vi "ShortcutMenu.vi"(8 "error in":errorcluster, 9 "menu ref in":refnum<k9>, 11 "node in":refnum<class "NISE_CEF_Node.lvclass">) -> (0 "error out":errorcluster, 1 "menu ref out":refnum<k9>, 3 "node out":refnum<class "NISE_CEF_Node.lvclass">)   [LabVIEW 2013, in "NISE_CEF_Node.lvclass"]
doc: "Defines the behavior of the shortcut menu of the node."
uses:
  NISE_CEF_Node.lvclass
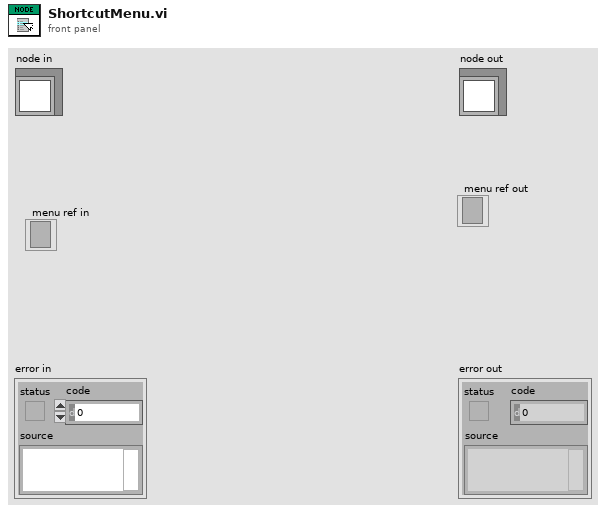
[diagram p1: front panel]
types:
  T1 = typedef "NISE_CEF_Node.lvclass/NodeMenuOptions.ctl" = cluster{"removable":bool, "movable":bool, "duplicate":bool}
  T2 = typedef "NISE_CEF_Node.lvclass/SubNodeCluster.ctl" = cluster{"subnodes menu name":string[], "subnodes class":string[]}
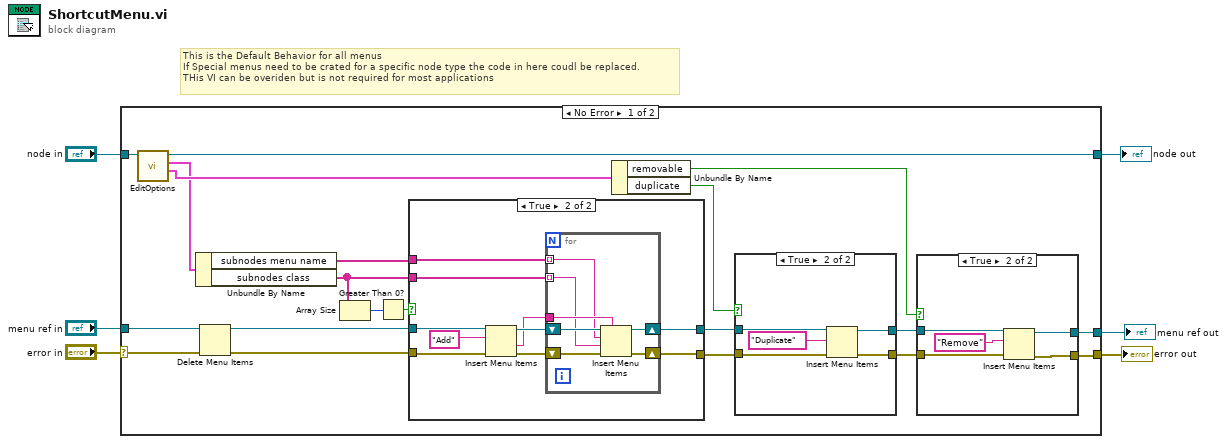
[diagram p0: block diagram]
diagram:
  # "This is the Default Behavior for all menus\nIf Special menus need to be crated for a specific node type the code in here coudl be replaced.\nTHis VI can be overiden but is not required for most applications"
  n1 = case shown="No Error" "error in" {
    selector: "error in" -> [w15 w61]
    tunnel: [w18 w62] -> w4
    tunnel: "node in" -> [w19 w62]
    tunnel: "menu ref in" -> [w20 w60]
    tunnel: [w13 w61] -> w2
    tunnel: [w7 w60] -> w1
    frame No Error {
      n2 = call-dynamic "EditOptions.vi"("node in"=w19) -> ("edit options"=w17:T1, "subnodes class"=w10:T2, "node out"=w18:refnum<class "NISE_CEF_Node.lvclass">)  [unwired: 7 in, 1 out]
      n3 = Unbundle By Name(w10) -> ("subnodes menu name"=w9:string[], "subnodes class"=w8:string[])
      n4 = Delete Menu Items(6:w15, 9:w20) -> (0:w23:errorcluster, 3:w24:refnum<k9>)  [unwired: 2 in]
      n5 = Array Size(array=w8) -> (size(s)=w26:i32)
      n6 = Greater Than 0?(x=w26) -> (x > 0?=w25:bool)
      n7 = case shown="True" w25 {
        tunnel: w24 -> [w42 w52]
        tunnel: w23 -> [w41 w51]
        tunnel: w9 -> [_ w46]
        tunnel: [w42 w45] -> w22
        tunnel: [w41 w44] -> w21
        tunnel: w8 -> [_ w43]
        frame False {
        }
        frame True {
          n8 = Insert Menu Items(6:w51, 8:"Add", 9:w52) -> (0:w48:errorcluster, 1:w47:string, 3:w49:refnum<k9>)  [unwired: 3 in]
          n9 = for {
            tunnel: w47 -> [w57]
            tunnel: w46 -> [w54] mode=indexing
            shift-right: [w56] -> w45
            shift-left: w49 -> [w59]
            shift-right: [w55] -> w44
            shift-left: w48 -> [w58]
            tunnel: w43 -> [w53] mode=indexing
            n10 = Insert Menu Items(5:w57, 6:w58, 7:w53, 8:w54, 9:w59) -> (0:w55:errorcluster, 3:w56:refnum<k9>)  [unwired: 1 in, 1 out]
          }
        }
      }
      n11 = Unbundle By Name(w17) -> ("removable"=w11:bool, "duplicate"=w16:bool)
      n12 = case shown="True" w16 {
        tunnel: w22 -> [w35 w40]
        tunnel: w21 -> [w34 w39]
        tunnel: [w35 w38] -> w12
        tunnel: [w34 w37] -> w14
        frame False {
        }
        frame True {
          n13 = Insert Menu Items(6:w39, 8:"Duplicate", 9:w40) -> (0:w37:errorcluster, 3:w38:refnum<k9>)  [unwired: 3 in, 1 out]
        }
      }
      n14 = case shown="True" w11 {
        tunnel: w14 -> [w28 w33]
        tunnel: [w28 w32] -> w13
        tunnel: w12 -> [w27 w31]
        tunnel: [w27 w29] -> w7
        frame False {
        }
        frame True {
          n15 = Insert Menu Items(6:w33, 8:"Remove", 9:w31) -> (0:w32:errorcluster, 3:w29:refnum<k9>)  [unwired: 3 in, 1 out]
        }
      }
    }
    frame Error {
    }
  }
  "error out" <- w2
  "node out" <- w4
  "menu ref out" <- w1
